vi "State_Machine.vi"(8 "error in (no error)":errorcluster caption="entrée d'erreur (pas d'erreur)", 11 "Wait_CloseFixture en entrée":refnum<class "Wait_CloseShielding.lvclass">) -> (0 "error out":errorcluster caption="sortie d'erreur", 2 "Json_String":string, 3 "Wait_CloseFixture en sortie":refnum<class "Wait_CloseShielding.lvclass">)   [LabVIEW 2020, in "Library Test.lvlib" / "Wait_CloseShielding.lvclass"]
uses:
  Wait_CloseShielding.lvclass
  C:/Users/ngarcin/OneDrive - Altyor/Standard TB/Class/Test/Test (Default)/Test (Default).lvclass
  Instrument/Instrument (Default)/Class Instrument (Default).lvclass
  Popup/Class Popup WaitShieldingBox/Class Popup WaitShieldingBox.lvclass
  C:/Users/ngarcin/OneDrive - Altyor/Standard TB/Class/Popup/Class Popup Operator_Validation/Class Popup Operator_Validation (Default)/Class Popup Operator_Validation (Virtual).lvclass
  C:/Users/ngarcin/OneDrive - Altyor/Standard TB/Class/Popup/Class Popup (Main)/Class Popup (Main).lvclass
  Wait_CloseShielding.lvclass/Wait_CloseShielding.ctl
  Commun VI/Library Commun.lvlib
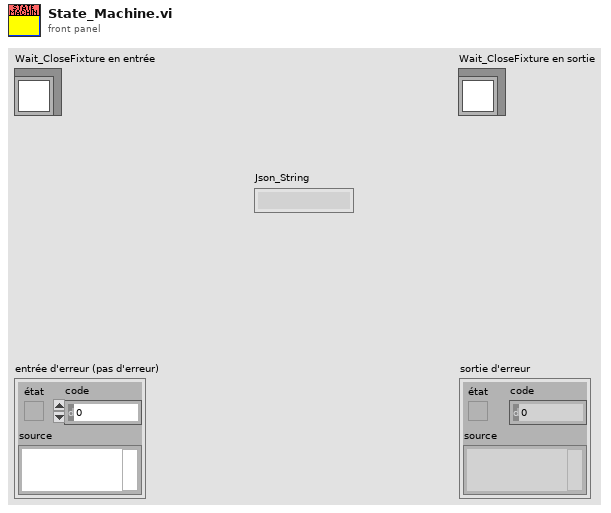
[diagram p1: front panel]
types:
  T1 = cluster{"Instrument Sheilding":refnum<class "Class Instrument (Default).lvclass">, "Timeout (ms)":u64, "Status Wait":enum16{"Erreur", "Close", "Open"}}
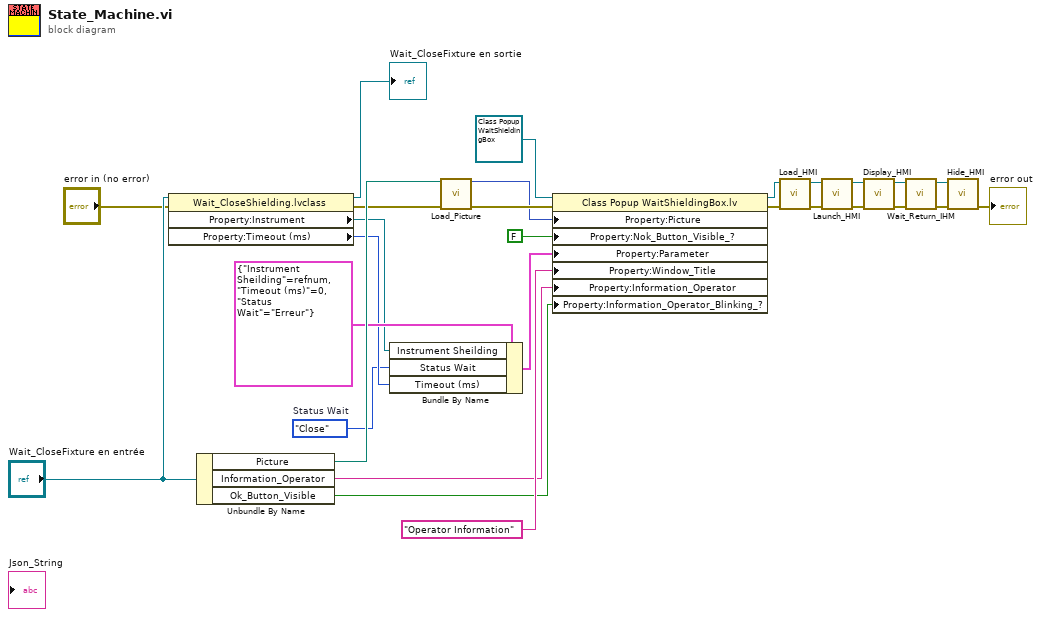
[diagram p0: block diagram]
diagram:
  w2 = enum16{"Erreur", "Close", "Open"}."Close"  # Status Wait
  n1 = property class="Wait_CloseShielding.lvclass"(reference="Wait_CloseFixture en entrée", error in="error in (no error)") -> (reference out=→"Wait_CloseFixture en sortie":refnum<class "Wait_CloseShielding.lvclass">, error out=w4:errorcluster, "Property:Instrument"=w6:refnum<class "Class Instrument (Default).lvclass">, "Property:Timeout (ms)"=w11:u64)
  n2 = Unbundle By Name("Wait_CloseFixture en entrée") -> ("Picture"=w20:path, "Information_Operator"=w23:string, "Ok_Button_Visible"=w22:bool)
  n3 = Bundle By Name(cluster=T1 {"Instrument Sheilding"=refnum, "Timeout (ms)"=0, "Status Wait"=enum."Erreur"}, "Instrument Sheilding"=w6, "Status Wait"=w2, "Timeout (ms)"=w11) -> (w3:T1)
  n4 = call "Load_Picture.vi"("Chemin In"=w20, "error in (no error)"=w4) -> ("Img Out"=w19:picture, "error out"=w21:errorcluster)  [unwired: 11 in, 1 out]
  n5 = property class="Class Popup WaitShieldingBox.lv"(reference=refnum<class "Class Popup WaitShieldingBox.lvclass"> refnum ("Library Popup.lvlib:Class Popup WaitShieldingBox.lvclass"), error in=w21, "Property:Picture"=w19, "Property:Nok_Button_Visible_?"=FALSE ("Nok_Button_Visible_?"), "Property:Parameter"=w3, "Property:Window_Title"="Operator Information" ("Window_Title"), "Property:Information_Operator"=w23, "Property:Information_Operator_Blinking_?"=w22) -> (reference out=w27:refnum<class "Class Popup WaitShieldingBox.lvclass">, error out=w26:errorcluster)
  n6 = call-dynamic "Load_HMI.vi"("error in (no error)"=w26, "Class Popup (Default) en entrée"=w27) -> ("error out"=w16:errorcluster, "Class Popup (Default) en sortie"=w17:refnum<class "Class Popup WaitShieldingBox.lvclass">)  [unwired: 8 in]
  n7 = call-dynamic "Launch_HMI.vi"("error in (no error)"=w16, "Class Popup (Default) en entrée"=w17) -> ("error out"=w28:errorcluster, "Class Popup (Default) en sortie"=w18:refnum<class "Class Popup WaitShieldingBox.lvclass">)  [unwired: 8 in]
  n8 = call-dynamic "Display_HMI.vi"("error in (no error)"=w28, "Class Popup (Default) en entrée"=w18) -> ("error out"=w10:errorcluster, "Class Popup (Default) en sortie"=w7:refnum<class "Class Popup WaitShieldingBox.lvclass">)  [unwired: 8 in]
  n9 = call-dynamic "Wait_Return_IHM.vi"("error in (no error)"=w10, "Class Popup (Default) en entrée"=w7) -> ("error out"=w9:errorcluster, "Class Popup (Default) en sortie"=w8:refnum<class "Class Popup WaitShieldingBox.lvclass">)  [unwired: 8 in]
  n10 = call-dynamic "Hide_HMI.vi"("error in (no error)"=w9, "Class Popup (Default) en entrée"=w8) -> ("error out"=→"error out":errorcluster)  [unwired: 8 in, 1 out]
